vi "Query Run Mode.vi"(8 "error in (no error)":errorcluster, 10 "Channel (0: Channel 1)":T1 items=["Channel 1", "Channel 2"], 11 "VISA resource name":refnum<visa-resource-name>) -> (0 "error out":errorcluster, 2 "Run Mode":u16(ring) items=["Continuous", "AM", "FM", "PM", "FSK", "PWM", "Sweep", "Burst"], 3 "VISA resource name out":refnum<visa-resource-name>)   [LabVIEW 2023, in "Tektronix AFG 3000 Series.lvlib"]
uses:
  Tektronix AFG 3000 Series.lvlib
  controls.llb/Channel.ctl
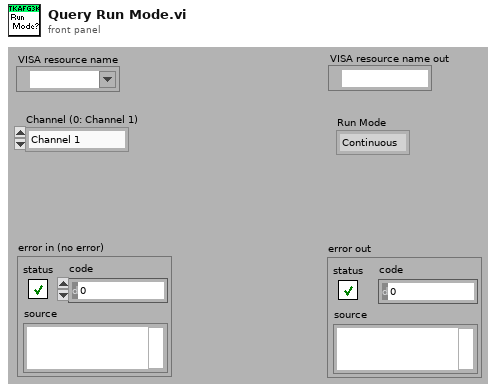
[diagram p1: front panel]
types:
  T1 = typedef "Channel.ctl" = u16
  T2 = typedef "Frequency Mode.ctl" = enum16{"CW", "Sweep"}
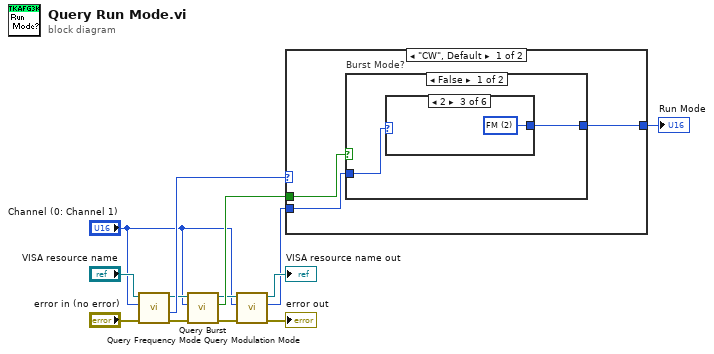
[diagram p0: block diagram]
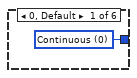
[diagram p2: hidden frame]
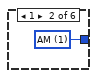
[diagram p3: hidden frame]
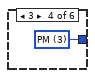
[diagram p4: hidden frame]
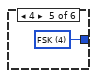
[diagram p5: hidden frame]
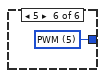
[diagram p6: hidden frame]
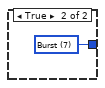
[diagram p7: hidden frame]
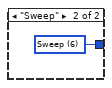
[diagram p8: hidden frame]
diagram:
  n1 = call "Query Frequency Mode.vi"("error in (no error)"="error in (no error)", "Channel (0: Channel 1)"="Channel (0: Channel 1)", "VISA resource name"="VISA resource name") -> ("error out"=w5:errorcluster, "Mode (0: CW)"=w11:T2, "VISA resource name out"=w8:refnum<visa-resource-name>)  [unwired: 6 out]
  n2 = call "Query Burst.vi"("error in (no error)"=w5, "Channel (0: Channel 1)"="Channel (0: Channel 1)", "VISA resource name"=w8) -> ("error out"=w4:errorcluster, "Burst Enabled?"=w9:bool, "VISA resource name out"=w7:refnum<visa-resource-name>)  [unwired: 6 out]
  n3 = call "Query Modulation Mode.vi"("error in (no error)"=w4, "Channel (0: Channel 1)"="Channel (0: Channel 1)", "VISA resource name"=w7) -> ("error out"=→"error out":errorcluster, "Modulation Mode"=w2:u16, "VISA resource name out"=→"VISA resource name out":refnum<visa-resource-name>)  [unwired: 6 out]
  n4 = case shown="\"CW\", Default" w11 {
    tunnel: [w15 w26] -> w10
    tunnel: w9 -> [w16 _]
    tunnel: w2 -> [w14 _]
    frame "CW", Default {
      n5 = case "Burst Mode?" shown="False" w16 {
        tunnel: [w17 w25] -> w15
        tunnel: w14 -> [w18 _]
        frame False {
          n6 = case shown="2" w18 {
            tunnel: [w19 w20 w21 w22 w23 w24] -> w17
            frame 0, Default {
              w19 = u16 0 items=["Continuous", "AM", "FM", "PM", "FSK", "PWM", "Sweep", "Burst"] ("Run Mode")
            }
            frame 1 {
              w20 = u16 1 items=["Continuous", "AM", "FM", "PM", "FSK", "PWM", "Sweep", "Burst"] ("Run Mode")
            }
            frame 2 {
              w21 = u16 2 items=["Continuous", "AM", "FM", "PM", "FSK", "PWM", "Sweep", "Burst"] ("Run Mode")
            }
            frame 3 {
              w22 = u16 3 items=["Continuous", "AM", "FM", "PM", "FSK", "PWM", "Sweep", "Burst"] ("Run Mode")
            }
            frame 4 {
              w23 = u16 4 items=["Continuous", "AM", "FM", "PM", "FSK", "PWM", "Sweep", "Burst"] ("Run Mode")
            }
            frame 5 {
              w24 = u16 5 items=["Continuous", "AM", "FM", "PM", "FSK", "PWM", "Sweep", "Burst"] ("Run Mode")
            }
          }
        }
        frame True {
          w25 = u16 7 items=["Continuous", "AM", "FM", "PM", "FSK", "PWM", "Sweep", "Burst"] ("Run Mode")
        }
      }
    }
    frame "Sweep" {
      w26 = u16 6 items=["Continuous", "AM", "FM", "PM", "FSK", "PWM", "Sweep", "Burst"] ("Run Mode")
    }
  }
  "Run Mode" <- w10
